vi "Update Task for Task Kind.vi"(9 "DAQmx Task":refnum<k21>, 10 "DAQmx Task prefix":string, 11 "Task Map in":map{string, refnum<k21>}(c390)) -> (3 "Task Map out":map{string, refnum<k21>}(c390))   [LabVIEW 2021, in "Load Frame.lvlib"]
uses:
  Load Frame.lvlib
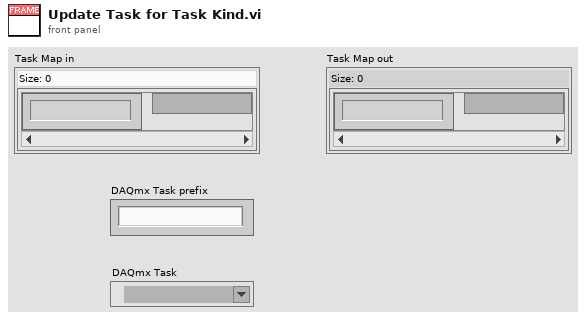
[diagram p1: front panel]
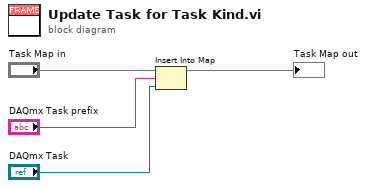
[diagram p0: block diagram]
diagram:
  n1 = Insert Into Map(map in="Task Map in", key="DAQmx Task prefix", value="DAQmx Task") -> (map out=→"Task Map out":map{string, refnum<k21>})  [unwired: 2 out]
